vi "RX-TX-BPCS-HMI-Modbus (SubVI).vi"(0 "Modbus Slave in":refnum<class "Modbus Slave.lvclass">, 5 "SIM-BPCS-RX-ARRAY":dbl[](array[numeric]), 7 "SIS-BPCS-RX-Array":bool[](array[boolean]), 9 "BPCS-SIM-TX-ARRAY":dbl[](array[numeric]), 11 "error in (no error)":errorcluster) -> (1 "HMI-10LIC200-KPID":dbl[](array[numeric]), 2 "HMI-10LIC200_MA":bool, 3 "HMI-10TIC100_MA":bool, 4 "Modbus Slave out":refnum<class "Modbus Slave.lvclass">, 6 "HMI-10LIC200-SP":dbl, 8 "HMI-10HIC200":dbl, 10 "HMI-10TIC100-SP":dbl, 12 "HMI-10HIC300":dbl, 13 "HMI-10HIC100":dbl, 14 "HMI-10TIC100-KPID":dbl[](array[numeric]), 15 "error out":errorcluster)   [LabVIEW 2018]
uses:
  <vilib>/Modbus/slave/Modbus Slave.lvclass
panel:
  out "register values":u16[](array[numeric])
  in  "Array in":dbl[](array[numeric])
  in  "type 2":u16[](array[numeric])
  in  "type":u16[](array[numeric])
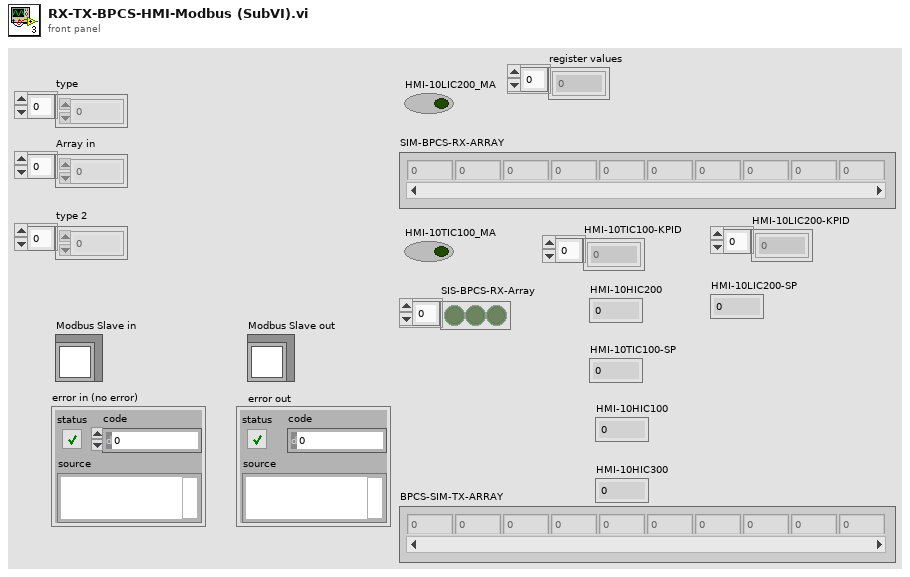
[diagram p1: front panel]
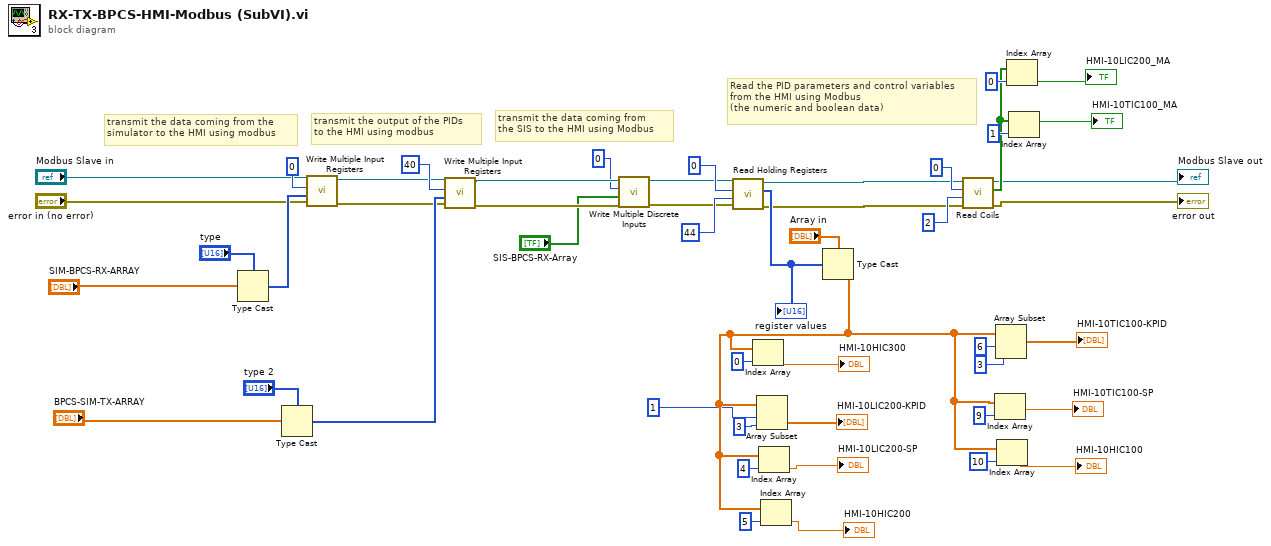
[diagram p0: block diagram]
diagram:
  # "Read the PID parameters and control variables \nfrom the HMI using Modbus\n(the numeric and boolean data)"
  # "transmit the data coming from \nthe SIS to the HMI using Modbus"
  # "transmit the output of the PIDs \nto the HMI using modbus"
  # "transmit the data coming from the \nsimulator to the HMI using modbus"
  n1 = Type Cast(type="type", x="SIM-BPCS-RX-ARRAY") -> (*(type *) &x=w8:u16[])
  n2 = Type Cast(type="type 2", x="BPCS-SIM-TX-ARRAY") -> (*(type *) &x=w16:u16[])
  n3 = call-dynamic "Write Multiple Input Registers.vi"("error in (no error)"="error in (no error)", "input register values"=w8, "starting address"=u16 0, "Modbus slave in"="Modbus Slave in") -> ("error out"=w10:errorcluster, "Modbus slave out"=w9:refnum<class "Modbus Slave.lvclass">)  [unwired: 6 in]
  n4 = call-dynamic "Write Multiple Input Registers.vi"("error in (no error)"=w10, "input register values"=w16, "starting address"=u16 40, "Modbus slave in"=w9) -> ("error out"=w12:errorcluster, "Modbus slave out"=w11:refnum<class "Modbus Slave.lvclass">)  [unwired: 6 in]
  n5 = call-dynamic "Write Multiple Discrete Inputs.vi"("error in (no error)"=w12, "discrete input values"="SIS-BPCS-RX-Array", "starting address"=u16 0, "Modbus slave in"=w11) -> ("error out"=w18:errorcluster, "Modbus slave out"=w17:refnum<class "Modbus Slave.lvclass">)  [unwired: 6 in]
  n6 = call-dynamic "Read Holding Registers.vi"("error in (no error)"=w18, "number of holding registers"=u16 44, "starting address"=u16 0, "Modbus slave in"=w17) -> ("error out"=w40:errorcluster, "register values"=w50:u16[], "Modbus slave out"=w39:refnum<class "Modbus Slave.lvclass">)  [unwired: 5 in]
  "register values" <- w50
  n7 = Type Cast(type="Array in", x=w50) -> (*(type *) &x=w35:dbl[])
  n8 = Index Array(array=w35, index=0) -> (element=→"HMI-10HIC300":dbl)
  n9 = Array Subset(array=w35, index=1, length=3) -> (→"HMI-10LIC200-KPID":dbl[])
  n10 = Index Array(array=w35, index=4) -> (element=→"HMI-10LIC200-SP":dbl)
  n11 = Index Array(array=w35, index=5) -> (element=→"HMI-10HIC200":dbl)
  n12 = call-dynamic "Read Coils.vi"("error in (no error)"=w40, "number of coils"=u16 2, "starting address"=u16 0, "Modbus slave in"=w39) -> ("error out"=→"error out":errorcluster, "coil values"=w45:bool[], "Modbus slave out"=→"Modbus Slave out":refnum<class "Modbus Slave.lvclass">)  [unwired: 5 in]
  n13 = Index Array(array=w35, index=9) -> (element=→"HMI-10TIC100-SP":dbl)
  n14 = Array Subset(array=w35, index=6, length=3) -> (→"HMI-10TIC100-KPID":dbl[])
  n15 = Index Array(array=w35, index=10) -> (element=→"HMI-10HIC100":dbl)
  n16 = Index Array(array=w45, index=0) -> (element=→"HMI-10LIC200_MA":bool)
  n17 = Index Array(array=w45, index=1) -> (element=→"HMI-10TIC100_MA":bool)
